vi "waveformformfile.vi"(2 "Matlab wave file":path, 3 "Sampling frequency (Hz)":dbl) -> (0 "wfsize":i32, 1 "Waveform":waveform(dbl))   [LabVIEW 2015]
uses:
  <vilib>/Utility/file.llb/Read Delimited Spreadsheet (DBL).vi
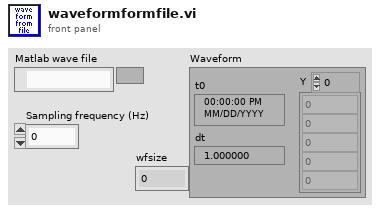
[diagram p1: front panel]
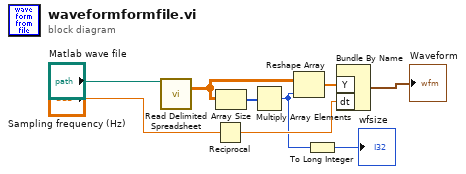
[diagram p0: block diagram]
diagram:
  n1 = call-poly <vilib>:"Read Delimited Spreadsheet.vi"("file path (dialog if empty)"="Matlab wave file") -> ("all rows"=w5:dbl[][])  [unwired: 9 in, 5 out]
  n2 = Reciprocal(x="Sampling frequency (Hz)") -> (1/x=w9:dbl)
  n3 = Array Size(array=w5) -> (size(s)=w6:i32[])
  n4 = Multiply Array Elements(1:w6) -> (0:w7:i32)
  n5 = Reshape Array(w5, w7) -> (w8:dbl[])
  n6 = To Long Integer(number=w7) -> (32bit integer=→"wfsize":i32)
  n7 = Bundle By Name("Y"=w8, "dt"=w9) -> (→"Waveform":waveform(dbl))  [unwired: 1 in]
